vi "Do.vi"(8 "error in (no error)":errorcluster, 10 "Actor in":refnum<class "Actor.lvclass">, 11 "Populate Menu Msg":refnum<class "Populate Menu Msg.lvclass">) -> (0 "error out":errorcluster, 2 "Actor out":refnum<class "Actor.lvclass">)   [LabVIEW 2017, in "Populate Menu Msg.lvclass"]
doc: "This VI delivers the message to the actor by calling the appropriate method(s) on the actor."
uses:
  <vilib>/gpm_packages/@cs/Test-executive-builder/Source/Test Executive Builder View/Test Executive Builder View Messages/Populate Menu Msg/Populate Menu Msg.lvclass
  <vilib>/ActorFramework/Actor/Actor.lvclass
  <vilib>/gpm_packages/@cs/Test-executive-builder/Source/Test Executive Builder View/Test Executive Builder View/Test Executive Builder View.lvclass
  C:/Program Files/National Instruments/LabVIEW 2017/vi.lib/ActorFramework/Actor/Actor.lvclass
  <vilib>/gpm_packages/@cs/Test-executive-builder/Source/Test Executive Builder View/Test Executive Builder View Messages/Populate Menu Msg/Populate Menu Msg.lvclass/Populate Menu Msg.ctl
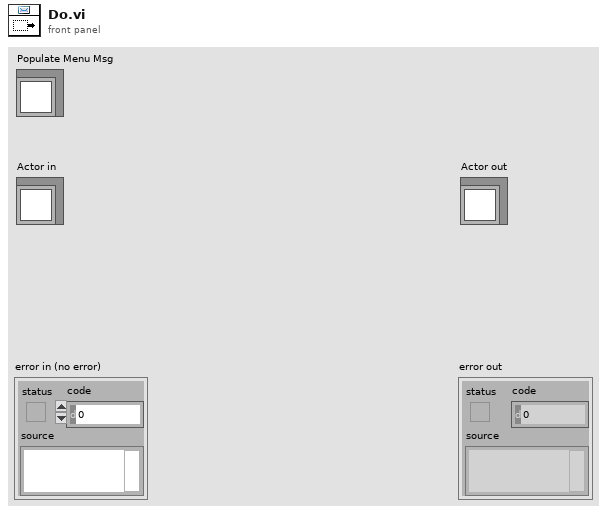
[diagram p1: front panel]
types:
  T1 = typedef "LVPoint32TypeDef.ctl" = cluster{"Horizontal":i32, "Vertical":i32}
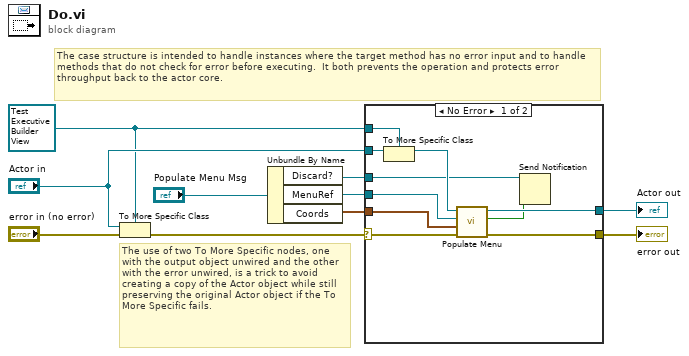
[diagram p0: block diagram]
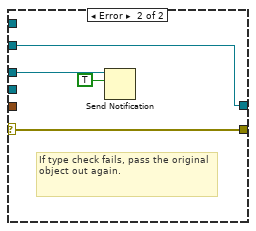
[diagram p2: hidden frame]
diagram:
  w4 = refnum<class "Test Executive Builder View.lvclass"> refnum ("Actor in")
  # "The use of two To More Specific nodes, one with the output object unwired and the other with the error unwired, is a trick to avoid creating a copy of the Actor object while still preserving the original Actor object if the To More Specific fails."
  # "The case structure is intended to handle instances where the target method has no error input and to handle methods that do not check for error before executing.  It both prevents the operation and protects error throughput back to the actor core."
  n1 = To More Specific Class(target class=w4, reference="Actor in", error in="error in (no error)") -> (error out=w8:errorcluster)  [unwired: 1 out]
  n2 = Unbundle By Name("Populate Menu Msg") -> ("Discard?"=w1:refnum<notifier>, "MenuRef"=w3:refnum<k9>, "Coords"=w2:T1)
  n3 = case shown="No Error" w8 {
    selector: w8 -> [w18 w24]
    tunnel: [w20 w24] -> w7
    tunnel: [w19 w23] -> w6
    tunnel: "Actor in" -> [w17 w23]
    tunnel: w4 -> [w16 _]
    tunnel: w3 -> [w14 _]
    tunnel: w2 -> [w13 _]
    tunnel: w1 -> [w12 w22]
    frame No Error {
      n4 = To More Specific Class(target class=w16, reference=w17) -> (specific class reference=w15:refnum<class "Test Executive Builder View.lvclass">)  [unwired: 1 in, 1 out]
      n5 = call-dynamic "Populate Menu.vi"("error in (no error)"=w18, "Coords"=w13, "MenuRef"=w14, "Test Executive Builder View in"=w15) -> ("error out"=w20:errorcluster, "Discard?"=w11:bool, "Test Executive Builder View out"=w19:refnum<class "Test Executive Builder View.lvclass">)  [unwired: 5 in]
      n6 = Send Notification(notification=w11, notifier=w12) -> ()  [unwired: 1 in, 2 out]
    }
    frame Error {
      # "If type check fails, pass the original object out again."
      n7 = Send Notification(notification=TRUE, notifier=w22) -> ()  [unwired: 1 in, 2 out]
    }
  }
  "error out" <- w7
  "Actor out" <- w6
